vi "FPGA_AIWriteOversampleBits.vi"(8 "error in (no error)":errorcluster, 9 "OversampleBit":u8, 10 "Channel":T1=enum."AI 1", 11 "AI Reference in":T2) -> (0 "error out":errorcluster, 3 "AI Reference out":T2)   [LabVIEW 2017]
uses:
  <vilib>/Rock Robotics/SystemInterfaces/AI/FPGA_AIDevRef.ctl
  <vilib>/Rock Robotics/SystemInterfaces/AI/FPGA_AIChannel.ctl
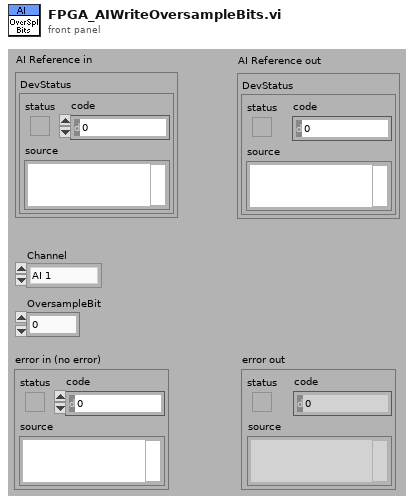
[diagram p1: front panel]
types:
  T1 = typedef "FPGA_AIChannel.ctl" = enum8{"AI 0", "AI 1", "AI 2", "AI 3", "AI MXP 0", "AI MXP 1", "AI MXP 2", "AI MXP 3", "Invalid"}
  T2 = typedef "FPGA_AIDevRef.ctl" = cluster{"DevStatus":errorcluster}
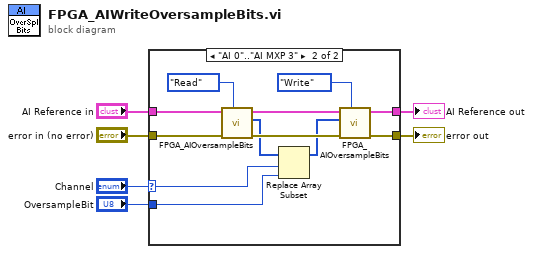
[diagram p0: block diagram]
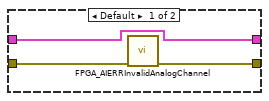
[diagram p2: hidden frame]
diagram:
  n1 = case shown="\"AI 0\"..\"AI MXP 3\"" "Channel" {
    selector: "Channel" -> [_ w21]
    tunnel: "OversampleBit" -> [_ w20]
    tunnel: [w9 w18] -> w4
    tunnel: "AI Reference in" -> [w9 w17]
    tunnel: "error in (no error)" -> [w8 w16]
    tunnel: [w7 w13] -> w1
    frame Default {
      n2 = call <vilib>:"FPGA_AIERRInvalidAnalogChannel.vi"("error in (no error)"=w8) -> ("error out"=w7:errorcluster)  [unwired: 10 in]
    }
    frame "AI 0".."AI MXP 3" {
      n3 = call <vilib>:"FPGA_AIOversampleBits.vi"("Task"=enum16{"Read", "Write"}."Read", "error in (no error)"=w16, "AI Reference in"=w17) -> ("error out"=w15:errorcluster, "OversampleBits out"=w12:u8[], "AI Reference out"=w19:T2)  [unwired: 1 in, 5 out]
      n4 = Replace Array Subset(array=w12, new element=w20, index=w21) -> (w14:u8[])
      n5 = call <vilib>:"FPGA_AIOversampleBits.vi"("Task"=enum16{"Read", "Write"}."Write", "error in (no error)"=w15, "OversampleBits in"=w14, "AI Reference in"=w19) -> ("error out"=w13:errorcluster, "AI Reference out"=w18:T2)  [unwired: 6 out]
    }
  }
  "AI Reference out" <- w4
  "error out" <- w1
